vi "Launch Action - DAQ AI Readers.vi"(7 "Init PackageID":i32, 8 "error in (no error)":errorcluster, 11 "DAQ AI Configurations":T1[](array[typedef]) {"Terminal Config" items=["Default"=-1, "RSE"=10083, "NRSE"=10078, "Differential"=10106, "Pseudodifferential"=12529]; "Min (V)" format="%#_13g"; "Max (V)" format="%#_13g"; "Sample Rate (Hz)" format="%#_13g"}) -> (0 "error out":errorcluster)   [LabVIEW 2021, in "XNET-CAN-Signal-Logger.lvlib"]
uses:
  XNET-CAN-Signal-Logger.lvlib
  Typedef/Def-DAQ AI Configuration.ctl
  Action - DAQ AI Reader.vi
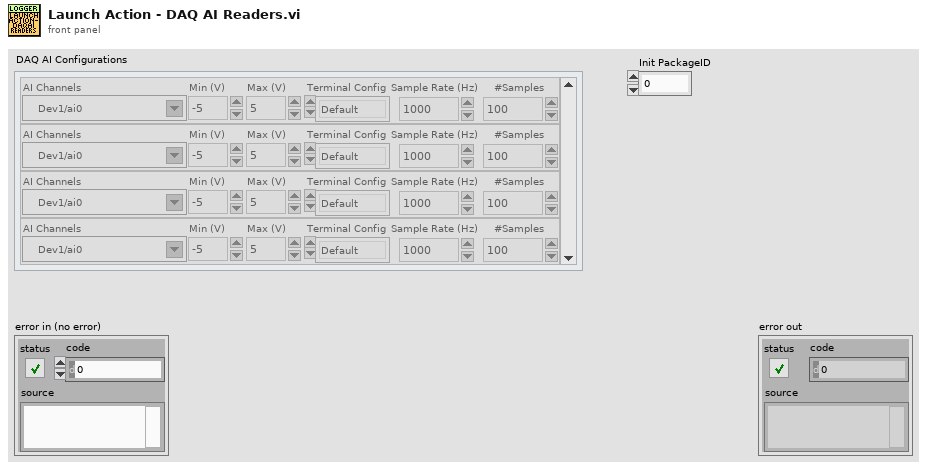
[diagram p1: front panel]
types:
  T1 = typedef "XNET-CAN-Signal-Logger.lvlib/Def-DAQ AI Configuration.ctl" = cluster{"AI Channels":tag, "Min (V)":dbl, "Max (V)":dbl, "Terminal Config":i32, "Sample Rate (Hz)":dbl, "#Samples":i32}
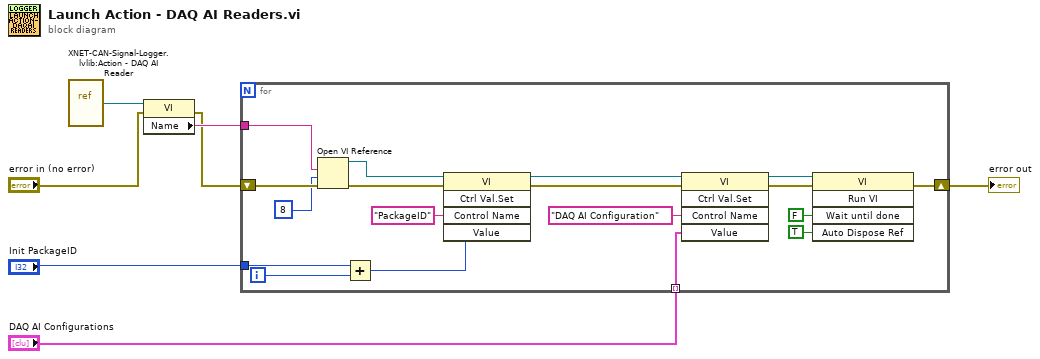
[diagram p0: block diagram]
diagram:
  n1 = vi-ref "XNET-CAN-Signal-Logger.lvlib:Action - DAQ AI Reader.vi"() -> (w7:refnum<vi>)
  n2 = property class="VI"(reference=w7, error in="error in (no error)") -> (error out=w4:errorcluster, "Name"=w6:string)  [unwired: 1 out]
  n3 = for {
    tunnel: w6 -> [w25]
    shift-right: [w18] -> w3
    shift-left: w4 -> [w23]
    tunnel: "DAQ AI Configurations" -> [w12] mode=indexing
    tunnel: "Init PackageID" -> [w8]
    i -> [w11]
    n4 = Open VI Reference(vi path=w25, options=8, error in (no error)=w23) -> (vi reference=w15:refnum<vi>, error out=w16:errorcluster)  [unwired: 3 in]
    n5 = Add(x=w8, y=w11) -> (x+y=w9:i32)
    n6 = invoke class="VI" method="Ctrl Val.Set"(reference=w15, error in=w16, "Control Name"="PackageID", "Value"=w9) -> (reference out=w14:refnum<vi>, error out=w13:errorcluster)  [unwired: 1 in, 3 out]
    n7 = invoke class="VI" method="Ctrl Val.Set"(reference=w14, error in=w13, "Control Name"="DAQ AI Configuration", "Value"=w12) -> (reference out=w22:refnum<vi>, error out=w21:errorcluster)  [unwired: 1 in, 3 out]
    n8 = invoke class="VI" method="Run VI"(reference=w22, error in=w21, "Wait until done"=FALSE ("Wait Until Done"), "Auto Dispose Ref"=TRUE ("Auto Dispose Reference")) -> (error out=w18:errorcluster)  [unwired: 1 in, 4 out]
  }
  "error out" <- w3
